vi "TANH Vector Elements.vi"(3 "X":T1) -> (14 "tanh(X)":T1)   [LabVIEW 2014]
uses:
  <vilib>/Analysis/Matrix/Datatypes/RealMatrix.ctl
  <vilib>/Analysis/Matrix/NI_Matrix.lvlib
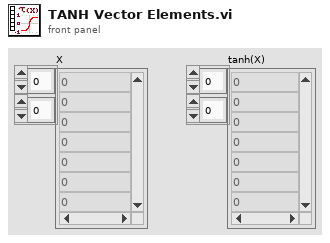
[diagram p1: front panel]
types:
  T1 = typedef "NI_Matrix.lvlib/RealMatrix.ctl" = dbl[][]
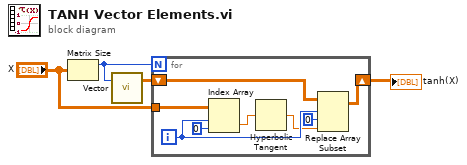
[diagram p0: block diagram]
diagram:
  n1 = Matrix Size(0:"X") -> (1:w3:i32)  [unwired: 1 out]
  n2 = call "Vector.vi"("length"=w3) -> ("Real Matrix (Column Vector)"=w2:T1)  [unwired: 18 in]
  n3 = for {
    N: w3 -> [_]
    tunnel: "X" -> [w9]
    shift-right: [w11] -> w1
    shift-left: w2 -> [w12]
    i -> [w8]
    n4 = Index Array(array=w9, index (row)=w8, index (col)=0) -> (element=w6:dbl)
    n5 = Hyperbolic Tangent(1:w6) -> (0:w5:dbl)
    n6 = Replace Array Subset(array=w12, new element=w5, index (row)=w8, index (col)=0 ("disabled index (col)")) -> (w11:T1)
  }
  "tanh(X)" <- w1
